vi "sv_Spectral Info for Harmonic Magnitude and Phase (N Channels).vi"(0 "channel info":T8[](array[typedef]) {"channel info"."pregain" format="%.2f"; "channel info"."weighting filter" items=["Linear", "A-weighting", "B-weighting", "C-weighting", "ITU-R 468-4", "Dolby", "CCITT", "C-message", "Wb", "Wc", "Wd", "We", "Wf", "Wh", "Wj", "Wk", "Wm", "AES17 20 kHz lowpass", "AES17 40 kHz lowpass", "AES17 20 kHz highpass", "AES17 40 kHz highpass"]; "channel info"."dB reference" format="%^.1e"; "channel info"."engineering units" items=["custom..."=0, "V"=1, "A"=21, "C"=30, "pC"=31, "s"=32, "-"=29, "Pa"=2, "N"=20, "g"=3, "m/s^2"=4, "m/s"=5, "m"=6, "mm/s"=12, "mm"=13, "micron/s"=14, "micron"=15, "in/s^2"=7, "in/s"=8, "in"=9, "mil/s"=10, "mil"=11, "rad/s^2"=16, "rad/s"=17, "rad"=18, "deg/s^2"=26, "deg/s"=27, "deg"=28, "RPM"=22, "cycle/s^2"=23, "Hz"=24, "cycle"=25, "strain"=19]; "channel info"."sensor sensitivity" format="%#_5f"}, 1 "reset? (T)":bool=TRUE, 7 "unit labels":string[](array[string]), 9 "orders to compute":dbl[](array[numeric]) format="%.2f", 11 "error in (no error)":errorcluster, 12 "view":T1={"dB on? (T)"=FALSE, "unwrap phase? (T)"=TRUE, "unit in degree? (T)"=TRUE}) -> (4 "spectrum info":T2[](array[typedef]) {"x-axis units" items=["Time (s)"=0, "Frequency-CB (Hz)"=1, "Frequency-CPB (Hz)"=1248, "Frequency-Arbitrary (Hz)"=2357, "Quefrency (s)"=2, "Revolutions (rev)"=3, "Order"=4, "Speed (RPM)"=11, "Speed (rad/s)"=21, "Index"=65535]; "weighting filter" items=["Linear", "A-weighting", "B-weighting", "C-weighting", "ITU-R 468-4", "Dolby", "CCITT", "C-message", "Wb", "Wc", "Wd", "We", "Wf", "Wh", "Wj", "Wk", "Wm", "AES17 20 kHz lowpass", "AES17 40 kHz lowpass", "AES17 20 kHz highpass", "AES17 40 kHz highpass"]; "dB reference [EU]" format="%.2f"; "engineering units" items=["custom..."=0, "V"=1, "A"=21, "C"=30, "pC"=31, "s"=32, "-"=29, "Pa"=2, "N"=20, "g"=3, "m/s^2"=4, "m/s"=5, "m"=6, "mm/s"=12, "mm"=13, "micron/s"=14, "micron"=15, "in/s^2"=7, "in/s"=8, "in"=9, "mil/s"=10, "mil"=11, "rad/s^2"=16, "rad/s"=17, "rad"=18, "deg/s^2"=26, "deg/s"=27, "deg"=28, "RPM"=22, "cycle/s^2"=23, "Hz"=24, "cycle"=25, "strain"=19]; "spectral info"."window" items=["None "=0, "Hanning"=1, "Hamming"=2, "Blackman-Harris"=3, "Exact Blackman"=4, "Blackman"=5, "Flat Top"=6, "4 Term B-Harris "=7, "7 Term B-Harris"=8, "Low Sidelobe"=9, "Force - Exponential"=10, "Gaussian"=62]}, 15 "error out":errorcluster)   [LabVIEW 2017, in "SoundVib_ContSweptSine.lvlib"]
uses:
  <vilib>/addons/Sound and Vibration/svt_Continuous Swept Sine/SoundVib_ContSweptSine.lvlib
  <vilib>/addons/_NISVFA/_Shared subVIs/Controls/svc_Resampled Channel Info.ctl
  <vilib>/addons/_NISVFA/_Shared subVIs/Controls/svc_Channel Info.ctl
  <vilib>/addons/_NISVFA/_Shared subVIs/Controls/svc_Engineering Units Text Ring.ctl
  <vilib>/addons/_NISVFA/_Shared subVIs/Controls/svc_Weighting Filter Text Ring.ctl
  <vilib>/addons/_NISVFA/_Shared subVIs/Controls/svc_Spectrum Info.ctl
  <vilib>/addons/_NISVFA/_Shared subVIs/Controls/svc_X-Axis Units.ctl
  <vilib>/addons/_NISVFA/_Shared subVIs/Controls/svc_Spectrum Type.ctl
  <vilib>/addons/_NISVFA/_Shared subVIs/Controls/svc_Complimentary Spectrum Units.ctl
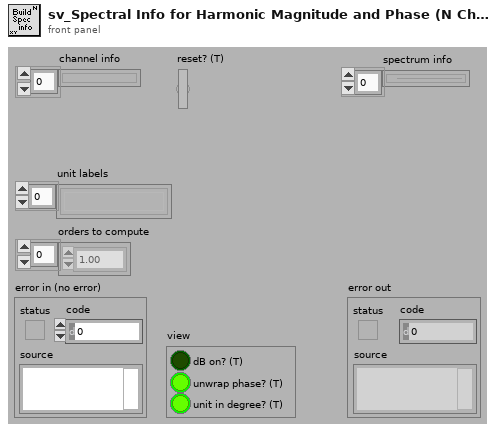
[diagram p1: front panel]
types:
  T1 = cluster{"dB on? (T)":bool, "unwrap phase? (T)":bool, "unit in degree? (T)":bool}
  T2 = typedef "svc_Spectrum Info.ctl" = cluster{"channel name":string, "description":string, "x-axis units":T3, "spectral info":cluster{"spectrum type":T4, "linear/dB":enum16{"linear", "dB"}, "window":u16, "window size":i32, "FFT size":i32}, "engineering units":T5, "custom label":string, "dB reference [EU]":dbl, "peak units":enum16{"rms", "peak", "peak-peak"}, "weighting filter":T6, "spectral density?":bool, "unit label":string, "spectrum skewed?":bool, "complimentary spectrum units":T7}
  T3 = typedef "svc_X-Axis Units.ctl" = u16
  T4 = typedef "svc_Spectrum Type.ctl" = enum16{"FFT Spectrum [complex]", "Amplitude [Magnitude]", "Power [Magnitude^2]", "Cross Spectrum [complex]", "Frequency Response [Complex]"}
  T5 = typedef "svc_Engineering Units Text Ring.ctl" = u16
  T6 = typedef "svc_Weighting Filter Text Ring.ctl" = u16
  T7 = typedef "svc_Complimentary Spectrum Units.ctl" = enum16{"none", "radians", "degrees", "cycles", "imaginary"}
  T8 = typedef "svc_Resampled Channel Info.ctl" = cluster{"channel name":string, "description":string, " channel info":T9}
  T9 = typedef "svc_Channel Info.ctl" = cluster{"sensor sensitivity":dbl, "engineering units":T5, "dB reference":dbl, "custom label":string, "weighting filter":T6, "pregain":dbl}
  T10 = cluster{"spectrum type":T4, "linear/dB":enum16{"linear", "dB"}, "window":u16, "window size":i32, "FFT size":i32}
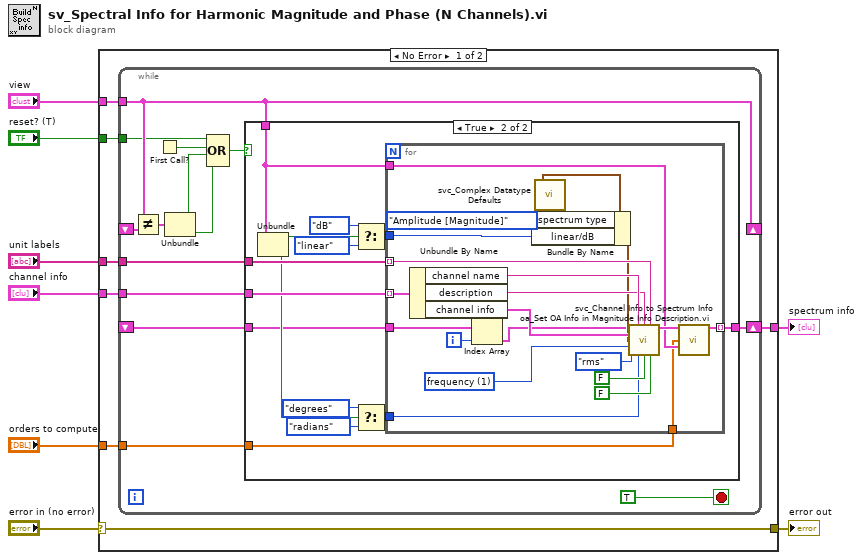
[diagram p0: block diagram]
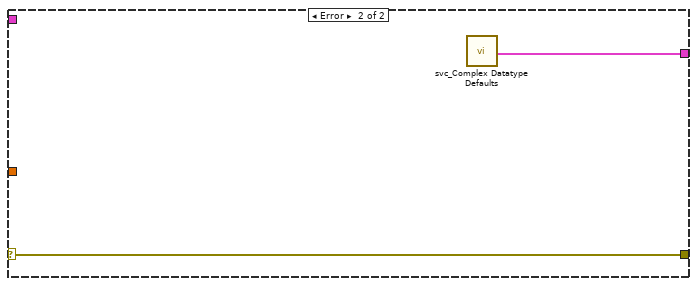
[diagram p3: hidden frame]
diagram:
  n1 = case shown="No Error" "error in (no error)" {
    selector: "error in (no error)" -> [w14 w67]
    tunnel: [w14 w67] -> w7
    tunnel: [w13 w66] -> w4
    tunnel: "channel info" -> [w15 _]
    tunnel: "unit labels" -> [w12 _]
    tunnel: "view" -> [w11 _]
    tunnel: "reset? (T)" -> [w10 _]
    tunnel: "orders to compute" -> [w9 _]
    frame No Error {
      n2 = while {
        tunnel: w15 -> [w29]
        tunnel: w12 -> [w27]
        shift-right: [w23] -> _
        shift-left: _ -> [w24]
        shift-right: [w28] -> w13
        shift-left: _ -> [w25]
        tunnel: w11 -> [w23]
        tunnel: w10 -> [w22]
        tunnel: w9 -> [w16]
        stop <- TRUE stop-if-true
        n3 = Not Equal?(x=w23, y=w24) -> (x != y?=w20:T1)
        n4 = First Call?() -> (First Call?: T/F=w21:bool)
        n5 = Unbundle(w20) -> ("dB on? (T)"=w19:bool, "unit in degree? (T)"=w18:bool)  [unwired: 1 out]
        n6 = Compound Arithmetic op=OR(w22, w21, w19, w18) -> (w17:bool)
        n7 = case shown="True" w17 {
          tunnel: w29 -> [_ w44]
          tunnel: [w30 w43] -> w28
          tunnel: w27 -> [_ w42]
          tunnel: w25 -> [w30 w33]
          tunnel: w23 -> [_ w32]
          tunnel: w16 -> [_ w31]
          frame False {
          }
          frame True {
            n8 = Unbundle(w32) -> ("dB on? (T)"=w38:bool, "unit in degree? (T)"=w37:bool)  [unwired: 1 out]
            n9 = Select(t=enum16{"linear", "dB"}."dB" ("spectral info.linear/dB"), s=w38, f=enum16{"linear", "dB"}."linear" ("spectral info.linear/dB")) -> (s? t:f=w39:enum16{"linear", "dB"})
            n10 = Select(t=svc_Complimentary_Spectrum_Units."degrees" ("complimentary spectrum units"), s=w37, f=svc_Complimentary_Spectrum_Units."radians" ("complimentary spectrum units")) -> (s? t:f=w34:T7)
            n11 = for {
              tunnel: w44 -> [w61] mode=indexing
              tunnel: [w47] -> w43 mode=indexing
              tunnel: w42 -> [w60] mode=indexing
              tunnel: w39 -> [w52]
              tunnel: w34 -> [w56]
              tunnel: w33 -> [w51]
              tunnel: w32 -> [w46]
              tunnel: w31 -> [w45]
              i -> [w50]
              w57 = u16 1 items=["time"=0, "frequency"=1, "quefrency"=2, "revolutions"=3, "order"=4, "rpm"=11] ("x-axis units")
              n12 = Unbundle By Name(w61) -> ("channel name"=w65:string, "description"=w64:string, "channel info"=w59:T9)
              n13 = Index Array(array=w51, index=w50) -> (element=w49:T2)
              n14 = call <vilib>:"svc_Complex Datatype Defaults.vi"() -> ("spectral info"=w55:T10)  [unwired: 11 in, 8 out]
              n15 = Bundle By Name(cluster=w55, "spectrum type"=svc_Spectrum_Type."Amplitude [Magnitude]", "linear/dB"=w52) -> (w54:T10)
              n16 = call <vilib>:"svc_Channel Info to Spectrum Info.vi"("spectrum info in"=w49, "channel name"=w65, "description"=w64, "unit label"=w60, "channel info"=w59, "spectral info"=w54, "x-axis units"=w57, "peak units"=enum16{"rms", "peak", "peak-peak"}."rms", "complimentary spectrum units"=w56, "spectral density?"=FALSE, "spectrum skewed?"=FALSE) -> ("spectrum info out"=w48:T2)  [unwired: 4 in]
              n17 = call <vilib>:"oa_Set OA Info in Magnitude Info Description.vi.vi"("magnitude info"=w48, "orders to compute"=w45, "view"=w46) -> ("magnitude info out"=w47:T2)  [unwired: 11 in, 1 out]
            }
          }
        }
      }
    }
    frame Error {
      n18 = call <vilib>:"svc_Complex Datatype Defaults.vi"() -> ("empty array of spectrum info"=w66:T2[])  [unwired: 11 in, 8 out]
    }
  }
  "error out" <- w7
  "spectrum info" <- w4
